vi "SelectErrorIndicatorType.vi"(1 "Error indicator type (primary)":T1, 12 "Error indicator type (secondary)":T1) -> (21 "Error indicator path":path)   [LabVIEW 2017, in "ErrorStructureDrawer.lvlib"]
doc: "Gets a path to the error indicator that corresponds to the type specified by \"Error indicator type (primary)\".\n\nIf the specified type is \"LabVIEW default\", then this VI will attempt to read the LabVIEW INI file to find out what the default type is. If that fails, or if the default type is not supported, then the VI will use the type specified by \"Error indicator type (secondary)\".\n\nIf the secondary choice is also \"LabVIEW default\", then the Modern type will be used."
uses:
  ErrorStructureDrawer.lvlib
  Controls/ErrorControlType.ctl
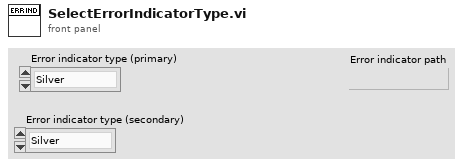
[diagram p1: front panel]
types:
  T1 = typedef "ErrorStructureDrawer.lvlib/ErrorControlType.ctl" = enum16{"Silver", "Modern", "Classic", "LabVIEW default"}
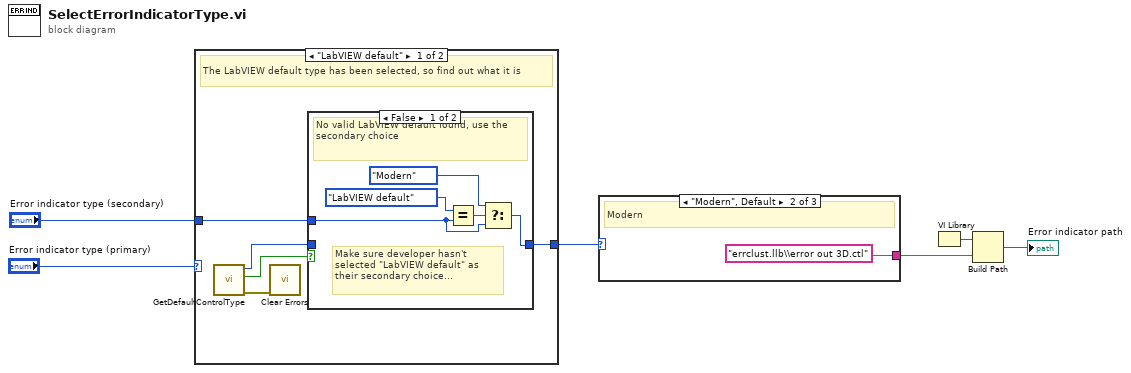
[diagram p0: block diagram]
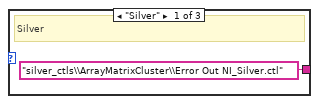
[diagram p4: hidden frame]
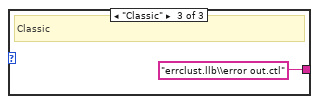
[diagram p5: hidden frame]
diagram:
  n1 = case shown="\"LabVIEW default\"" "Error indicator type (primary)" {
    selector: "Error indicator type (primary)" -> [_ w18]
    tunnel: [w7 w18] -> w4
    tunnel: "Error indicator type (secondary)" -> [w8 _]
    frame "LabVIEW default" {
      # "The LabVIEW default type has been selected, so find out what it is"
      n2 = call "GetDefaultControlType.vi"() -> ("Error Out"=w11:errorcluster, "Default control style valid?"=w10:bool, "Error control type"=w9:T1)  [unwired: 9 in]
      n3 = call <vilib>:"Clear Errors.vi"("error in (no error)"=w11) -> ()  [unwired: 5 in, 2 out]
      n4 = case shown="False" w10 {
        tunnel: w9 -> [_ w17]
        tunnel: w8 -> [w13 _]
        tunnel: [w14 w17] -> w7
        frame False {
          # "Make sure developer hasn't selected \"LabVIEW default\" as their secondary choice..."
          # "No valid LabVIEW default found, use the secondary choice"
          n5 = Equal?(x=ErrorControlType."LabVIEW default" ("Error control type (secondary)"), y=w13) -> (x = y?=w15:bool)
          n6 = Select(t=ErrorControlType."Modern" ("Error control type (secondary)"), s=w15, f=w13) -> (s? t:f=w14:T1)
        }
        frame True {
          # "Valid LabVIEW default found - use it"
        }
      }
    }
    frame "Modern", Default {
      # "A type has been specified directly, so use it"
    }
  }
  n7 = case shown="\"Modern\", Default" w4 {
    tunnel: ["silver_ctls\\ArrayMatrixCluster\\Error Out NI_Silver.ctl" ("name or relative path") "errclust.llb\\error out 3D.ctl" ("name or relative path") "errclust.llb\\error out.ctl" ("name or relative path")] -> w3
    frame "Silver" {
      # "Silver"
    }
    frame "Modern", Default {
      # "Modern"
    }
    frame "Classic" {
      # "Classic"
    }
  }
  n8 = VI Library() -> (path=w6:path)
  n9 = Build Path(base path=w6, name or relative path=w3) -> (appended path=→"Error indicator path":path)
